vi "Save Image.vi"(8 "error in (no error)":errorcluster, 10 "Paths":path[](array[path]), 11 "ImageHandler in":refnum<class "ImageHandler.lvclass">) -> (0 "error out":errorcluster, 3 "ImageHandler out":refnum<class "ImageHandler.lvclass">)   [LabVIEW 2022 SP3, in "ImageHandler.lvlib" / "ImageHandler.lvclass"]
uses:
  ImageHandler.lvclass
  C:/Program Files/National Instruments/LabVIEW 2022/vi.lib/ActorFramework/Actor/Actor.lvclass
  <vilib>/ActorFramework/Actor/Actor.lvclass/Actor.ctl
  ImageHandler - Controller -- Interface/ImageHandler - Controller -- Interface Messages/Acquisition Status Msg/Acquisition Status Msg.lvclass/Acquisition Status Msg.ctl
  <vilib>/ActorFramework/Message Enqueuer/Message Enqueuer.lvclass/Message Enqueuer.ctl
  <vilib>/ActorFramework/Message Enqueuer/Enqueue.vi
  ImageHandler - Controller -- Interface/ImageHandler - Controller -- Interface Messages/Acquisition Status Msg/Acquisition Status Msg.lvclass
  C:/Program Files/National Instruments/LabVIEW 2022/vi.lib/ActorFramework/Message/Message.lvclass
  <vilib>/ActorFramework/Message Priority Queue/Priority Enqueue.vi
  <vilib>/ActorFramework/Actor/Actor.lvclass
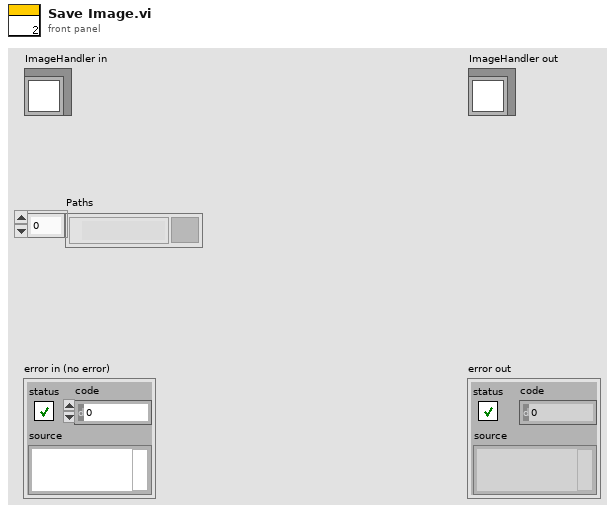
[diagram p1: front panel]
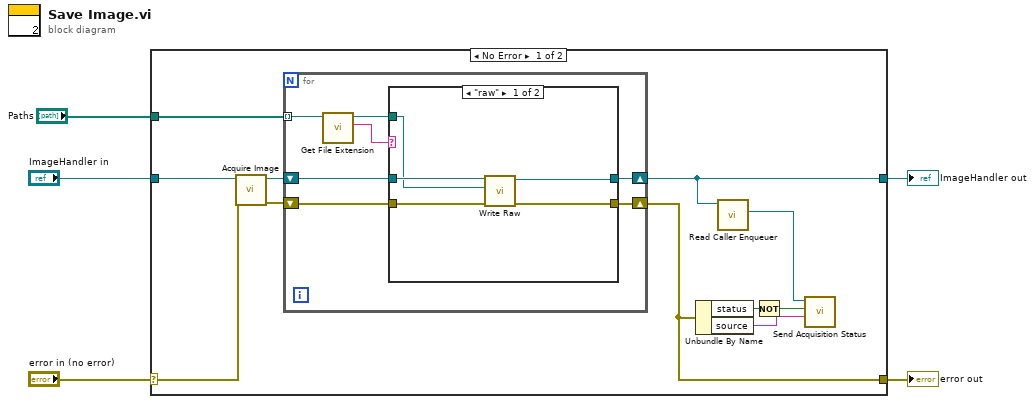
[diagram p0: block diagram]
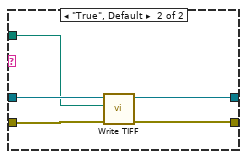
[diagram p2: hidden frame]
diagram:
  n1 = case shown="No Error" "error in (no error)" {
    selector: "error in (no error)" -> [w16 w35]
    tunnel: [w9 w35] -> w4
    tunnel: [w11 w34] -> w2
    tunnel: "ImageHandler in" -> [w14 w34]
    tunnel: "Paths" -> [w12 _]
    frame No Error {
      n2 = call "Acquire Image.vi"("error in (no error)"=w16, "ImageHandler in"=w14) -> ("error out"=w15:errorcluster, "ImageHandler out"=w13:refnum<class "ImageHandler.lvclass">)  [unwired: 8 in]
      n3 = for {
        tunnel: w12 -> [w19] mode=indexing
        shift-right: [w22] -> w9
        shift-left: w15 -> [w21]
        shift-right: [w23] -> w11
        shift-left: w13 -> [w20]
        n4 = call <vilib>:"Get File Extension.vi"("file"=w19) -> ("lowercase file extension"=w17:string, "dup file"=w18:path)  [unwired: 6 in, 3 out]
        n5 = case shown="\"raw\"" w17 {
          tunnel: w20 -> [w28 w33]
          tunnel: [w27 w32] -> w23
          tunnel: w21 -> [w26 w31]
          tunnel: [w25 w30] -> w22
          tunnel: w18 -> [w24 w29]
          frame "raw" {
            n6 = call "Write Raw.vi"("error in (no error)"=w26, "Path"=w24, "ImageHandler in"=w28) -> ("error out"=w25:errorcluster, "ImageHandler out"=w27:refnum<class "ImageHandler.lvclass">)  [unwired: 7 in]
          }
          frame "True", Default {
            n7 = call "Write TIFF.vi"("error in (no error)"=w31, "Path"=w29, "ImageHandler in"=w33) -> ("error out"=w30:errorcluster, "ImageHandler out"=w32:refnum<class "ImageHandler.lvclass">)  [unwired: 7 in]
          }
        }
      }
      n8 = Unbundle By Name(w9) -> ("status"=w8:bool, "source"=w7:string)
      n9 = call <vilib>:"Read Caller Enqueuer.vi"("Actor"=w11) -> ("Caller Enqueuer"=w10:refnum<class "Message Enqueuer.lvclass">)  [unwired: 10 in]
      n10 = Not(x=w8) -> (.not. x?=w6:bool)
      n11 = call "Send Acquisition Status.vi"("Remarks"=w7, "Status"=w6, "Message Enqueuer"=w10) -> ()  [unwired: 7 in, 2 out]
    }
    frame Error {
    }
  }
  "error out" <- w4
  "ImageHandler out" <- w2
